vi "python intergation test.vi"() -> ()   [LabVIEW 2023]
panel:
  out "Destination":dbl[][](array[numeric])
  out "error out":errorcluster
  out "Image Pixels (U8)":u8[][](array[numeric])
  out "Image Pixels (Float)":sgl[][](array[numeric]) format="%.2f"
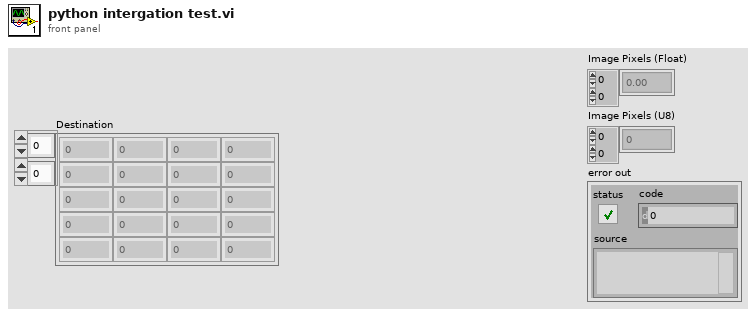
[diagram p1: front panel]
types:
  T1 = typedef "Image Type" = u32
  T2 = typedef "IMAQ Image.ctl" = refnum<image>
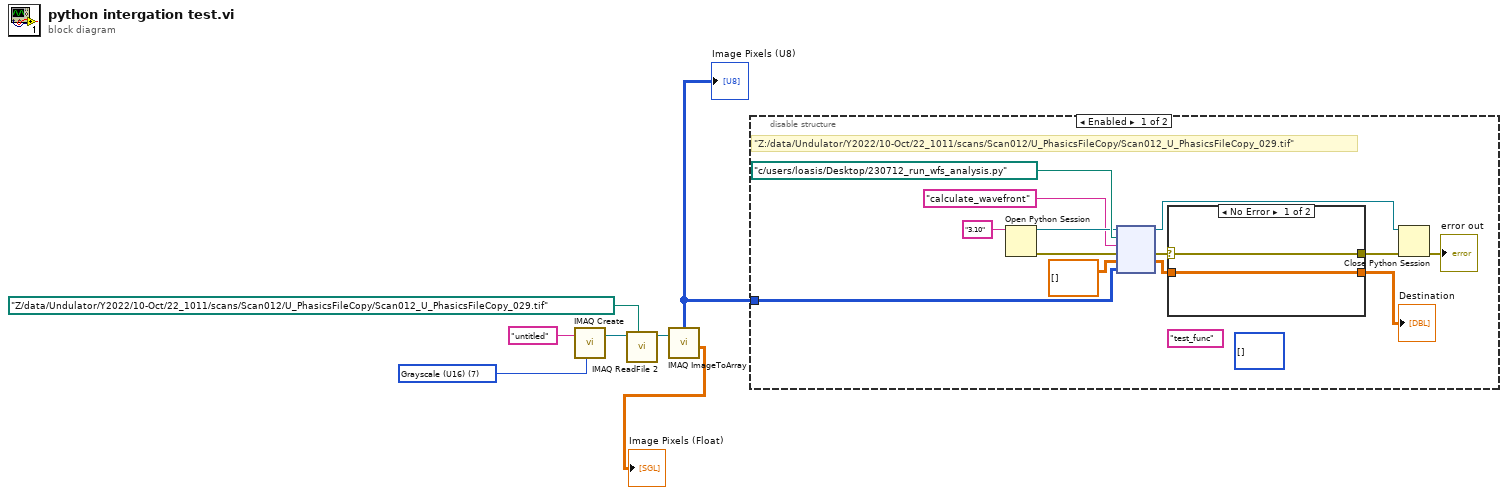
[diagram p0: block diagram]
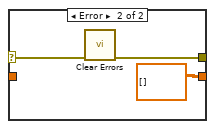
[diagram p2: hidden frame]
diagram:
  w6 = T1 7 items=["Grayscale (U8)", "Grayscale (I16)", "Grayscale (SGL)", "Complex (CSG)", "RGB (U32)", "HSL (U32)", "RGB (U64)", "Grayscale (U16)"] ("Image Type")
  n1 = call "IMAQ Create"("Image Name"="untitled", "Image Type"=w6) -> ("New Image"=w5:T2)  [unwired: 3 in, 1 out]
  n2 = call "IMAQ ReadFile 2"("File Path"=path "Z:/data/Undulator/Y2022/10-Oct/22_1011/scans/Scan012/U_PhasicsFileCopy/Scan012_U_PhasicsFileCopy_029.tif" ("module path"), "Image"=w5) -> ("Image Out"=w3:T2)  [unwired: 5 in, 4 out]
  n3 = call "IMAQ ImageToArray"("Image"=w3) -> ("Image Pixels (Float)"=→"Image Pixels (Float)":sgl[][], "Image Pixels (U8)"=w1:u8[][])  [unwired: 3 in, 3 out]
  "Image Pixels (U8)" <- w1
  n4 = disable-structure shown="Enabled" {
    disable-tunnel: w1 -> [w16 _]
    frame Enabled {
      (unwired) i32[][] [] ("Destination")
      (unwired) "test_func" ("function name")
      # "\"Z:/data/Undulator/Y2022/10-Oct/22_1011/scans/Scan012/U_PhasicsFileCopy/Scan012_U_PhasicsFileCopy_029.tif\""
      n5 = Open Python Session(python version="3.10" ("Python version")) -> (session out=w18:refnum<k35>, error out=w15:errorcluster)  [unwired: 2 in]
      n6 = node(w18, path "c:/users/loasis/Desktop/230712_run_wfs_analysis.py" ("module path"), "calculate_wavefront" ("function name"), w15, dbl[][] [] ("Destination"), w16) -> (w14:refnum<k35>, w17:errorcluster, w8:dbl[][])  [unwired: 1 in, 2 out]
      n7 = case shown="No Error" w17 {
        selector: w17 -> [w22 w25]
        tunnel: [w21 dbl[][] [] ("Destination")] -> w10
        tunnel: [w22 w24] -> w12
        tunnel: w8 -> [w21 _]
        frame No Error {
        }
        frame Error {
          n8 = call <vilib>:"Clear Errors.vi"("error in (no error)"=w25) -> ("error out"=w24:errorcluster)  [unwired: 5 in, 1 out]
        }
      }
      "Destination" <- w10
      n9 = Close Python Session(session in=w14, error in=w12) -> (11:→"error out":errorcluster)
    }
    frame Disabled {
    }
  }
